vi "Temperature Warnings.vi"() -> ()   [LabVIEW 2014]
doc: "在本练习中，将输入和输出放置在簇中。"
panel:
  out "气象数据输出":T1={"当前温度"=0.0, "最高温度"=0.0, "最低温度"=0.0, "警告？"=FALSE, "警告文本"="无警告"}
  in  "气象数据输入":T1={"当前温度"=0.0, "最高温度"=0.0, "最低温度"=0.0, "警告？"=FALSE, "警告文本"="无警告"}
  out "错误输出":cluster{"状态":bool, "代码":i32, "源":string}
  in  "错误输入":cluster{"状态":bool, "代码":i32, "源":string}
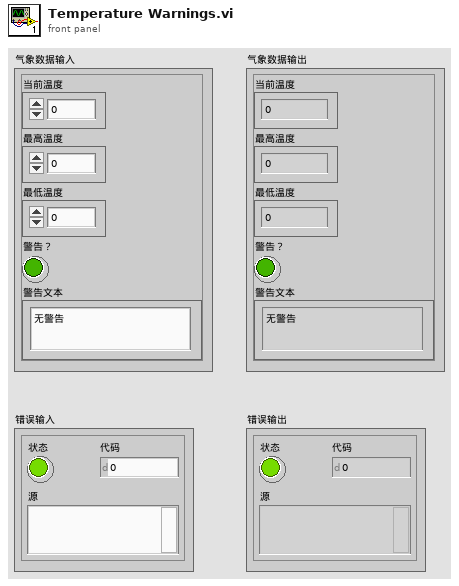
[diagram p1: front panel]
types:
  T1 = cluster{"当前温度":dbl, "最高温度":dbl, "最低温度":dbl, "警告？":bool, "警告文本":string}
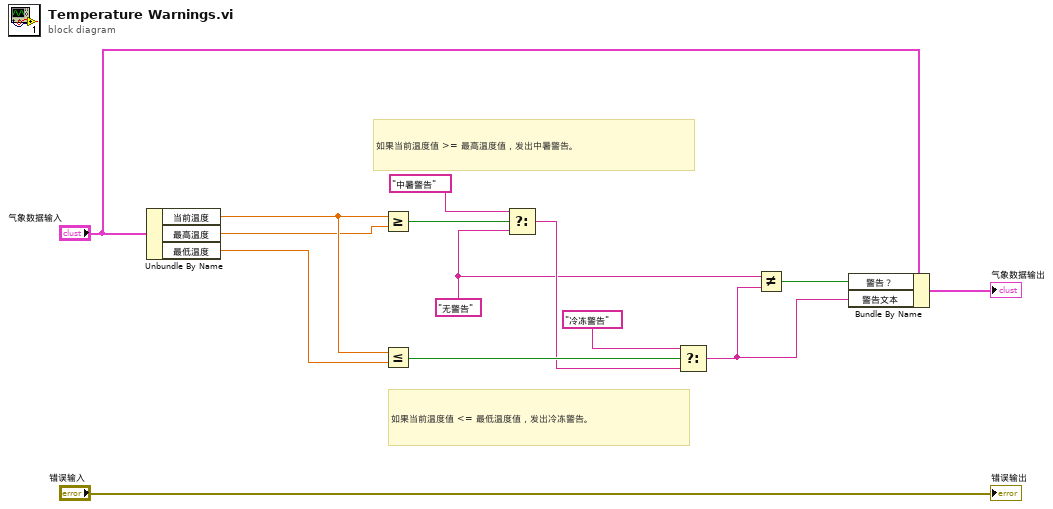
[diagram p0: block diagram]
diagram:
  w1 = "无警告" ("f")
  # "如果当前温度值 <= 最低温度值，发出冷冻警告。"
  # "如果当前温度值 >= 最高温度值，发出中暑警告。"
  n1 = Unbundle By Name("气象数据输入") -> ("当前温度"=w13:dbl, "最高温度"=w12:dbl, "最低温度"=w11:dbl)
  n2 = Greater Or Equal?(x=w13, y=w12) -> (x >= y?=w6:bool)
  n3 = Less Or Equal?(x=w13, y=w11) -> (x <= y?=w3:bool)
  n4 = Select(t="中暑警告", s=w6, f=w1) -> (s? t:f=w2:string)
  n5 = Select(t="冷冻警告", s=w3, f=w2) -> (s? t:f=w10:string)
  n6 = Not Equal?(x=w1, y=w10) -> (x != y?=w9:bool)
  n7 = Bundle By Name(cluster="气象数据输入", "警告？"=w9, "警告文本"=w10) -> (→"气象数据输出":T1)
  "错误输出" <- "错误输入"
